vi "Reset.vi"(8 "error in (no error)":errorcluster, 11 "Debug Latest Message in":refnum<class "Debug Latest Message.lvclass">) -> (0 "error out":errorcluster, 3 "Debug Latest Message out":refnum<class "Debug Latest Message.lvclass">)   [LabVIEW 2020, in "Debug Latest Message.lvclass"]
uses:
  Debug Latest Message.lvclass
  Debug Latest Message.lvclass/Debug Latest Message.ctl
  Debug Data/Debug Data.lvclass
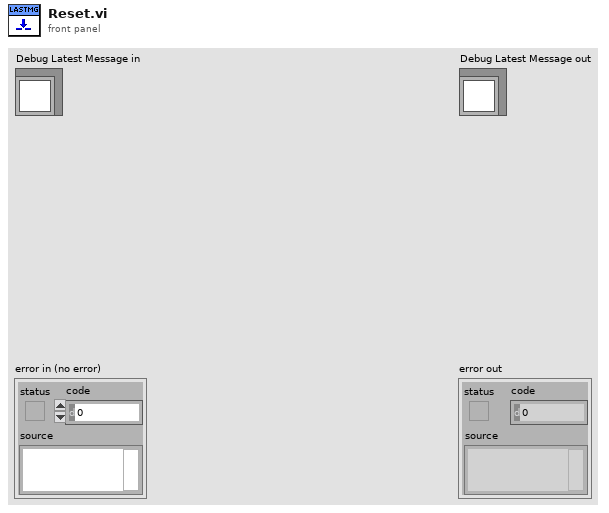
[diagram p1: front panel]
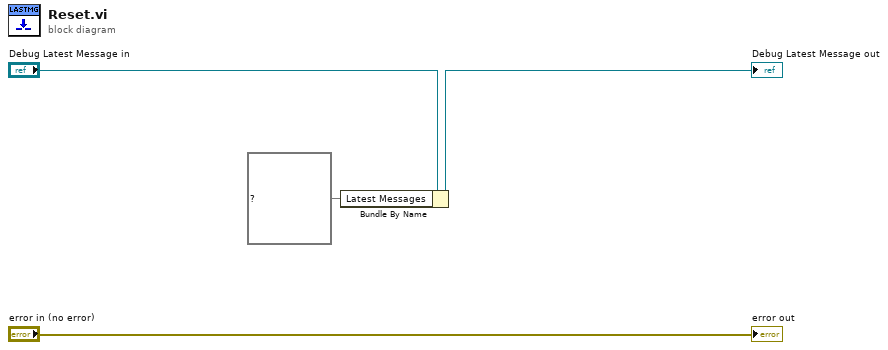
[diagram p0: block diagram]
diagram:
  n1 = Bundle By Name(cluster="Debug Latest Message in", "Latest Messages"=map{string, refnum<class "Debug Data.lvclass">} {}) -> (→"Debug Latest Message out":refnum<class "Debug Latest Message.lvclass">)
  "error out" <- "error in (no error)"
